vi "Construct (Array).vi"(8 "Error in (no error)":errorcluster, 10 "Priorities":T1[](array[typedef]) items=["EMERGENCY", "ALERT", "CRITICAL", "ERROR", "WARNING", "NOTICE", "INFO", "DEBUG"], 11 "LogFilterPriority in":refnum<class "LogFilterPriority.lvclass">) -> (0 "Error out":errorcluster, 3 "LogFilterPriority out":refnum<class "LogFilterPriority.lvclass">)   [LabVIEW 2011, in "LogFilterPriority.lvclass"]
uses:
  LogFilterPriority.lvclass
  Log/PrioritiesRing.ctl
  LogFilterPriority.lvclass/LogFilterPriority.ctl
  Log/Log.lvclass
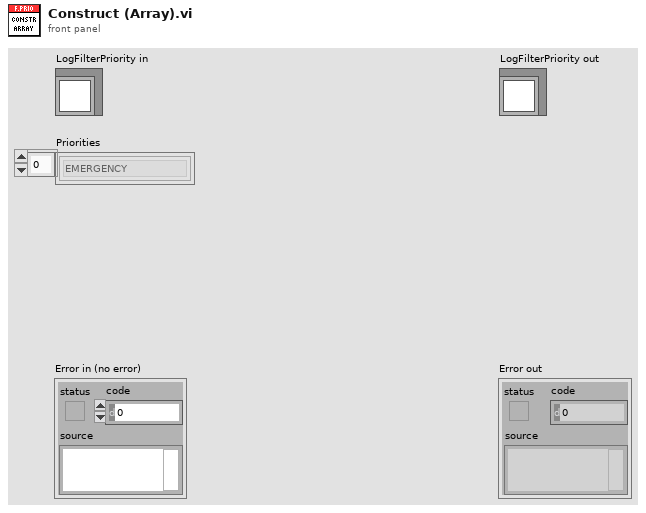
[diagram p1: front panel]
types:
  T1 = typedef "Log.lvclass/PrioritiesRing.ctl" = u32
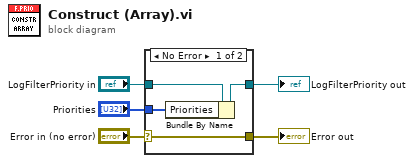
[diagram p0: block diagram]
diagram:
  n1 = case shown="No Error" "Error in (no error)" {
    selector: "Error in (no error)" -> [w9 w10]
    tunnel: [w9 w10] -> w4
    tunnel: [w7 w11] -> w2
    tunnel: "LogFilterPriority in" -> [w8 w11]
    tunnel: "Priorities" -> [w6 _]
    frame No Error {
      n2 = Bundle By Name(cluster=w8, "Priorities"=w6) -> (w7:refnum<class "LogFilterPriority.lvclass">)
    }
    frame Error {
    }
  }
  "Error out" <- w4
  "LogFilterPriority out" <- w2
